vi "host.orderbook.tester.vi"(8 "error in":errorcluster, 9 "Execute?":bool=TRUE, 10 "Seconds to Wait":i32=10, 11 "OrderBook.Command[]\nto Send":T4[](array[typedef])=[{"OrderBook Command.Type"=enum."AddOrder", "Side (U8)"=66, "Order Id (U64)"=0, "Quantity (U32)"=125, "Symbol (U64)"=29033, "Price (U64)"=9811, "Executed Quantity (U32)"=0, "Cancelled Quantity (U32)"=0}, {"OrderBook Command.Type"=enum."Get.All.Orders", "Side (U8)"=66, "Order Id (U64)"=0, "Quantity (U32)"=0, "Symbol (U64)"=29033, "Price (U64)"=0, "Executed Quantity (U32)"=0, "Cancelled Quantity (U32)"=0}] {"Side (U8)" format="%.0x"; "Order Id (U64)" format="%.0x"; "Symbol (U64)" format="%.0x"}) -> (0 "error out":errorcluster, 2 "OrderBook.Variables":T1, 3 "OrderBook.Entries":T2[](array[typedef]))   [LabVIEW 2020]
uses:
  arty/orderbook/orderbook.command.ctl
  arty/orderbook/orderbook.command.type.ctl
  arty/application/orderbook.entry.ctl
  arty/application/orderbook.result.type.ctl
  <vilib>/rvi/interface/RandomDataEmulation/nirviRandomDataOpen.vi
  <vilib>/rvi/interface/RandomDataEmulation/niFpgaWriteControlTemplate.vi
  <vilib>/rvi/interface/RandomDataEmulation/nirviRandomDataDMAMethods.vi
  <vilib>/rvi/interface/RandomDataEmulation/niFpgaReadControlTemplate.vi
  <vilib>/rvi/interface/RandomDataEmulation/nirviRandomDataClose.vi
  <vilib>/rvi/interface/nirviOpenFPGA/nirviOpenFPGA.xnode
  arty/orderbook/orderbook.test.vi
  <vilib>/rvi/interface/nirviReadWriteControl/nirviReadWriteControl.xnode
  <vilib>/rvi/interface/nirviMethod/nirviMethod.xnode
  <vilib>/rvi/interface/nirviCloseFPGA/nirviCloseFPGA.xnode
panel:
  out "Results.size":i32
  out "Results":u64[](array[numeric])
  out "Data.size":i32=8
  out "Data":u64[](array[numeric])=[0, 66, 0, 125, 29033, 9811, 0, 0] format="%.0x"
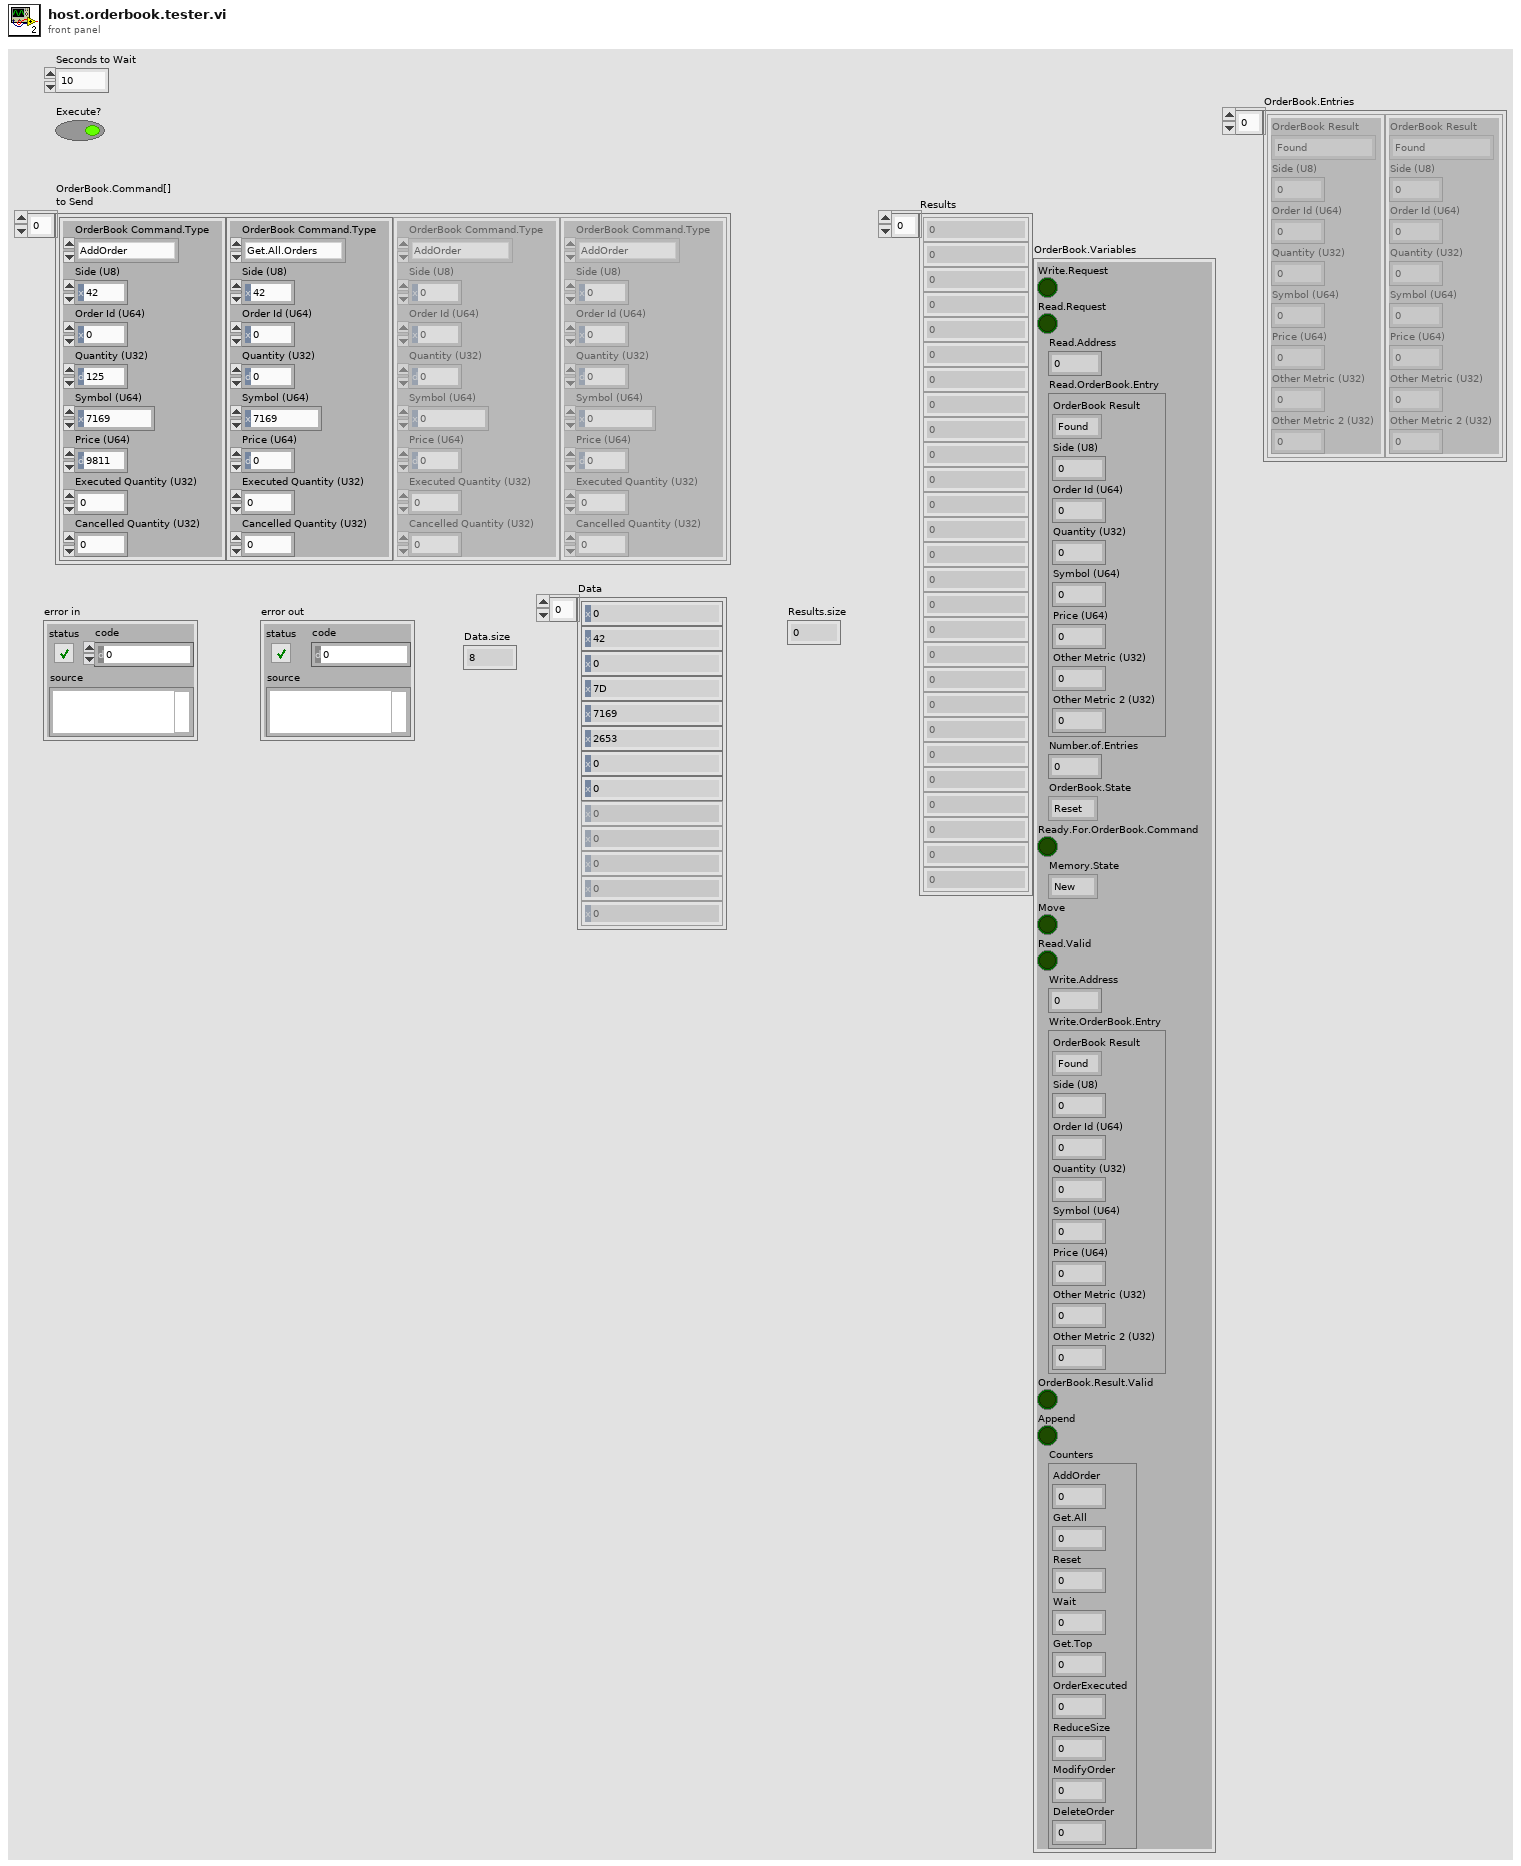
[diagram p1: front panel]
types:
  T1 = cluster{"Write.Request":bool, "Read.Request":bool, "Read.Address":u32, "Read.OrderBook.Entry":cluster{"OrderBook Result":enum16{"Found", "Not.Found"}, "Side (U8)":u8, "Order Id (U64)":u64, "Quantity (U32)":u32, "Symbol (U64)":u64, "Price (U64)":u64, "Other Metric (U32)":u32, "Other Metric 2 (U32)":u32}, "Number.of.Entries":u32, "OrderBook.State":enum16{"Reset", "Wait", "Get.Top", "Get.All.Orders", "AddOrder", "Order.Executed", "Reduce.Size", "Modify.Order", "Delete.Order"}, "Ready.For.OrderBook.Command":bool, "Memory.State":enum16{"New", "Request.Data", "Append", "Data.Ready"}, "Move":bool, "Read.Valid":bool, "Write.Address":u32, "Write.OrderBook.Entry":cluster{"OrderBook Result":enum16{"Found", "Not.Found"}, "Side (U8)":u8, "Order Id (U64)":u64, "Quantity (U32)":u32, "Symbol (U64)":u64, "Price (U64)":u64, "Other Metric (U32)":u32, "Other Metric 2 (U32)":u32}, "OrderBook.Result.Valid":bool, "Append":bool, "Counters":cluster{"AddOrder":u32, "Get.All":u32, "Reset":u32, "Wait":u32, "Get.Top":u32, "OrderExecuted":u32, "ReduceSize":u32, "ModifyOrder":u32, "DeleteOrder":u32}}
  T2 = typedef "orderbook.entry.ctl" = cluster{"OrderBook Result":T3, "Side (U8)":u8, "Order Id (U64)":u64, "Quantity (U32)":u32, "Symbol (U64)":u64, "Price (U64)":u64, "Other Metric (U32)":u32, "Other Metric 2 (U32)":u32}
  T3 = typedef "orderbook.result.type.ctl" = enum16{"Found", "Not.Found"}
  T4 = typedef "orderbook.command.ctl" = cluster{"OrderBook Command.Type":T5, "Side (U8)":u8, "Order Id (U64)":u64, "Quantity (U32)":u32, "Symbol (U64)":u64, "Price (U64)":u64, "Executed Quantity (U32)":u32, "Cancelled Quantity (U32)":u32}
  T5 = typedef "orderbook.command.type.ctl" = enum16{"AddOrder", "OrderExecuted", "ReduceSize", "ModifyOrder", "DeleteOrder", "Get.All.Orders", "Get.Top"}
  T6 = cluster{"Write.Request":bool, "Read.Request":bool, "Read.Address":u32, "Read.OrderBook.Entry":cluster{"OrderBook Result":enum16{"Found", "Not.Found"}, "Side (U8)":u8, "Order Id (U64)":u64, "Quantity (U32)":u32, "Symbol (U64)":u64, "Price (U64)":u64, "Other Metric (U32)":u32, "Other Metric 2 (U32)":u32}, "Number.of.Entries":u32, "OrderBook.State":enum16{"Reset", "Wait", "Get.Top", "Get.All.Orders", "AddOrder", "Order.Executed", "Reduce.Size", "Modify.Order", "Delete.Order"}, "Ready.For.OrderBook.Command":bool, "Memory.State":enum16{"New", "Request.Data", "Append", "Data.Ready"}, "Move":bool, "Read.Valid":bool, "Write.Address":u32, "Write.OrderBook.Entry":cluster{"OrderBook Result":enum16{"Found", "Not.Found"}, "Side (U8)":u8, "Order Id (U64)":u64, "Quantity (U32)":u32, "Symbol (U64)":u64, "Price (U64)":u64, "Other Metric (U32)":u32, "Other Metric 2 (U32)":u32}, "OrderBook.Result.Valid":bool, "Append":bool, "Counters":cluster{"Add":u32, "Get.All":u32, "Reset":u32, "Wait":u32, "Get.Top":u32, "Executed":u32, "ReduceSize":u32, "Modify":u32, "Delete":u32}}
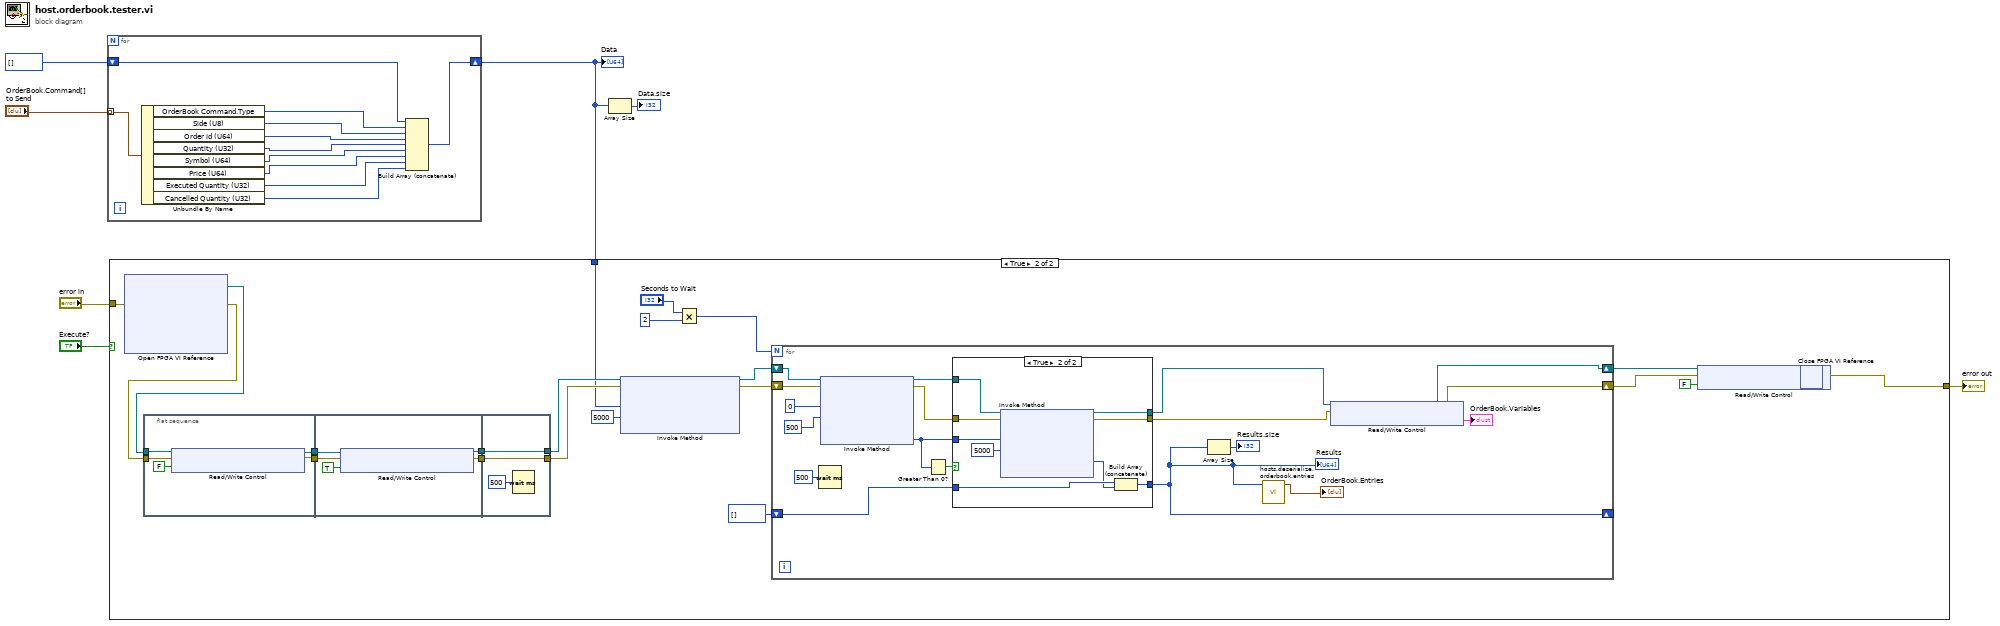
[diagram p0: block diagram]
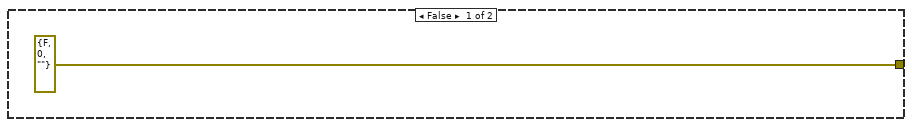
[diagram p2: hidden frame]
diagram:
  n1 = for {
    tunnel: "OrderBook.Command[]\nto Send" -> [w18] mode=indexing
    shift-right: [w9] -> w1
    shift-left: u64[] [] ("DataIn") -> [w8]
    n2 = Unbundle By Name(w18) -> ("OrderBook Command.Type"=w17:T5, "Side (U8)"=w16:u8, "Order Id (U64)"=w15:u64, "Quantity (U32)"=w14:u32, "Symbol (U64)"=w13:u64, "Price (U64)"=w12:u64, "Executed Quantity (U32)"=w11:u32, "Cancelled Quantity (U32)"=w10:u32)
    n3 = Build Array (concatenate)(w8, w17, w16, w15, w14, w13, w12, w11, w10) -> (w9:u64[])
  }
  "Data" <- w1
  n4 = case shown="True" "Execute?" {
    tunnel: [errorcluster {"status"=FALSE, "code"=0, "source"=""} ("error out") w20] -> w7
    tunnel: "error in" -> [_ w32]
    tunnel: w1 -> [_ w29]
    frame False {
    }
    frame True {
      n5 = xnode "Open FPGA VI Reference"("error in"=w32) -> ("FPGA VI Reference Out"=w25:refnum<k20>, "error out"=w24:errorcluster)  [unwired: 1 in]
      n6 = flat-sequence {
        tunnel: w25 -> [w43]
        tunnel: w24 -> [w44]
        tunnel: [w45] -> w36
        tunnel: [w46] -> w35
        tunnel: [w50] -> w38
        tunnel: [w49] -> w37
        tunnel: w36 -> [w48]
        tunnel: w35 -> [w47]
        tunnel: w38 -> [w52]
        tunnel: w37 -> [w53]
        tunnel: [w53] -> w31
        tunnel: [w52] -> w30
        frame #0 {
          n7 = xnode "Read/Write Control"("FPGA VI Reference In"=w43, "error in"=w44, "Reset"=FALSE ("reset")) -> ("FPGA VI Reference Out"=w46:refnum<k20>, "error out"=w45:errorcluster)
        }
        frame #1 {
          n8 = xnode "Read/Write Control"("FPGA VI Reference In"=w47, "error in"=w48, "Reset"=TRUE ("reset")) -> ("FPGA VI Reference Out"=w49:refnum<k20>, "error out"=w50:errorcluster)
        }
        frame #2 {
          n9 = Wait (ms)(milliseconds to wait=u32 500) -> ()  [unwired: 1 out]
        }
      }
      n10 = xnode "Invoke Method"("FPGA VI Reference In"=w31, "error in"=w30, "Data"=w29, "Timeout (ms)"=5000) -> ("FPGA VI Reference Out"=w41:refnum<k20>, "error out"=w40:errorcluster)  [unwired: 1 out]
      n11 = Multiply(x="Seconds to Wait", y=2) -> (x*y=w28:i32)
      n12 = for {
        N: w28 -> [_]
        shift-right: [w57] -> _
        shift-left: u64[] [] -> [w65]
        shift-right: [w60] -> w26
        shift-left: w41 -> [w72]
        shift-right: [w59] -> w21
        shift-left: w40 -> [w71]
        n13 = Wait (ms)(milliseconds to wait=u32 500) -> ()  [unwired: 1 out]
        n14 = xnode "Invoke Method"("FPGA VI Reference In"=w72, "error in"=w71, "Number of Elements"=u32 0, "Timeout (ms)"=500) -> ("FPGA VI Reference Out"=w66:refnum<k20>, "error out"=w64:errorcluster, "Elements Remaining"=w67:u32)  [unwired: 1 out]
        n15 = Greater Than 0?(x=w67) -> (x > 0?=w68:bool)
        n16 = case shown="True" w68 {
          tunnel: w67 -> [_ w84]
          tunnel: w66 -> [w74 w82]
          tunnel: [w75 w79] -> w57
          tunnel: w65 -> [w75 w81]
          tunnel: [w74 w78] -> w61
          tunnel: [w73 w77] -> w58
          tunnel: w64 -> [w73 w76]
          frame False {
          }
          frame True {
            n17 = xnode "Invoke Method"("FPGA VI Reference In"=w82, "error in"=w76, "Number of Elements"=w84, "Timeout (ms)"=5000) -> ("FPGA VI Reference Out"=w78:refnum<k20>, "error out"=w77:errorcluster, "Data"=w80:u64[])  [unwired: 1 out]
            n18 = Build Array (concatenate)(w81, w80) -> (w79:u64[])
          }
        }
        "Results" <- w57
        n19 = Array Size(array=w57) -> (size(s)=→"Results.size":i32)
        n20 = call "hosts.deserialize.orderbook.entries.vi"("DataIn"=w57) -> ("OrderBook.Entries"=→"OrderBook.Entries":T2[])  [unwired: 10 in]
        n21 = xnode "Read/Write Control"("FPGA VI Reference In"=w61, "error in"=w58) -> ("FPGA VI Reference Out"=w60:refnum<k20>, "error out"=w59:errorcluster, "OrderBook.Variables"=→"OrderBook.Variables":T6)
      }
      n22 = xnode "Read/Write Control"("FPGA VI Reference In"=w26, "error in"=w21, "Reset"=FALSE) -> ("FPGA VI Reference Out"=w23:refnum<k20>, "error out"=w20:errorcluster)
      n23 = xnode "Close FPGA VI Reference"("FPGA VI Reference In"=w23) -> ()  [unwired: 1 in, 1 out]
    }
  }
  "error out" <- w7
  n24 = Array Size(array=w1) -> (size(s)=→"Data.size":i32)
